vi "Agilent 33XXX Series Generate Arbitrary Waveform.vi"() -> ()   [LabVIEW 2012]
doc: "Shows how to configure then create an arbitrary waveform."
uses:
  Instance           2 56Saved   Agilent 33XXX Series Generate Arbitrary Waveform .vi
  Instance           1 56Saved   Agilent 33XXX Series Generate Arbitrary Waveform .vi
  <instrlib>/Agilent 33XXX Series/Agilent 33XXX Series.lvlib
panel:
  in  "Serial Configuration":T1={"Baud Rate"=9600, "Parity"=0, "Data Bits"=8, "Flow Control"=4} {"Flow Control" items=["None", "XON/XOFF", "RTS/CTS", "XON/XOFF & RTS/CTS", "DTR/DSR", "XON/XOFF & DTR/DSR"]; "Data Bits" items=["7"=7, "8"=8]; "Parity" items=["None", "Odd", "Even", "Mark", "Space"]; "Baud Rate" items=["300"=300, "600"=600, "1200"=1200, "2400"=2400, "4800"=4800, "9600"=9600, "19200"=19200]}
  in  "VISA resource name":refnum<visa-resource-name>
  in  "Frequency (1000 Hz)":dbl=1000.0
  in  "Gain (1.0)":dbl=1.0
  in  "Offset (0 V)":dbl
  in  "Arbitrary Waveform Name":string="ARB1"
  # "(c) 2005 - 2013 National Instruments.  ALL RIGHTS RESERVED."
  # "To edit the Arbitrary Waveform, use the Simulate Arbitrary Signal on the block diagram."
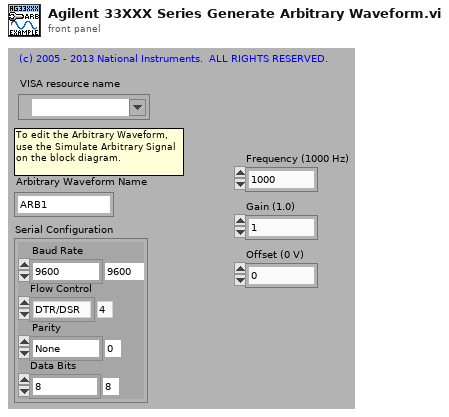
[diagram p1: front panel]
types:
  T1 = cluster{"Baud Rate":u32, "Parity":u16, "Data Bits":u16, "Flow Control":u16}
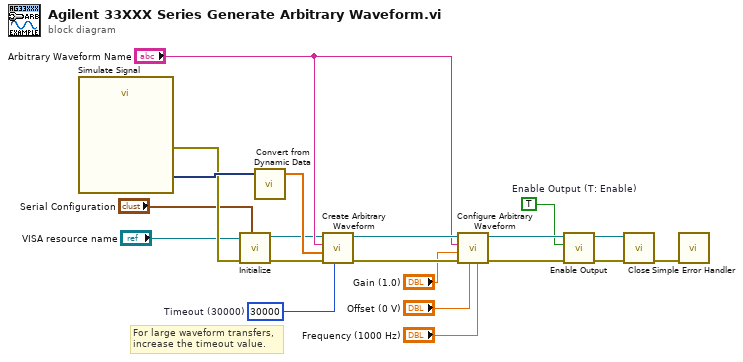
[diagram p0: block diagram]
diagram:
  w9 = u32 30000  # Timeout (30000)
  w13 = TRUE  # Enable Output (T: Enable)
  # "For large waveform transfers, increase the timeout value."
  n1 = call "Simulate Signal"() -> ("Sine with Uniform Noise"=w6:dynamicdata, "error out"=w4:errorcluster)  [unwired: 14 in]
  n2 = call <instrlib>:"Initialize.vi"("Serial Configuration"="Serial Configuration", "error in (no error)"=w4, "VISA resource name"="VISA resource name") -> ("error out"=w5:errorcluster, "VISA resource name out"=w7:refnum<visa-resource-name>)  [unwired: 7 in]
  n3 = call "Convert from Dynamic Data"("Dynamic Data Type"=w6) -> ("Array"=w8:dbl[])  [unwired: 3 in]
  n4 = call <instrlib>:"Create Arbitrary Waveform.vi"("Timeout (10000)"=w9, "error in (no error)"=w5, "Arbitrary Waveform Data"=w8, "Arbitrary Waveform Name (\"ARB1\")"="Arbitrary Waveform Name", "VISA resource name"=w7) -> ("error out"=w18:errorcluster, "VISA resource name out"=w19:refnum<visa-resource-name>)  [unwired: 5 in]
  n5 = call <instrlib>:"Configure Arbitrary Waveform.vi"("Frequency (1000 Hz)"="Frequency (1000 Hz)", "Offset (0.00 V)"="Offset (0 V)", "error in (no error)"=w18, "Gain (1.0)"="Gain (1.0)", "Arbitrary Waveform Name (\"ARB1\")"="Arbitrary Waveform Name", "VISA resource name"=w19) -> ("error out"=w16:errorcluster, "VISA resource name out"=w17:refnum<visa-resource-name>)  [unwired: 4 in]
  n6 = call <instrlib>:"Enable Output.vi"("error in (no error)"=w16, "Enable Output  (T: Enable)"=w13, "VISA resource name"=w17) -> ("error out"=w15:errorcluster, "VISA resource name out"=w14:refnum<visa-resource-name>)  [unwired: 7 in]
  n7 = call <instrlib>:"Close.vi"("error in (no error)"=w15, "VISA resource name"=w14) -> ("error out"=w20:errorcluster)  [unwired: 9 in]
  n8 = call <vilib>:"Simple Error Handler.vi"("error in (no error)"=w20) -> ()  [unwired: 4 in, 5 out]
